vi "SMTP Email Command.vi"(4 "error in (no error)":errorcluster, 6 "command":string, 7 "smtp session":T1) -> (0 "error out":errorcluster, 1 "reply":string, 2 "reply code":i32, 3 "smtp session out":T1)   [LabVIEW 2011, in "NewNI_SMTPEmail.lvlib"]
doc: "General pupose VI that sends any kind of message (command) to the SMTP server using \"SMTP Session\", and recieves a string of reply (possibly multiline as specified in RFC821)."
uses:
  NewNI_SMTPEmail.lvlib
  SMTP Email Session.ctl
panel:
  in  "tcp connection":refnum<k5>
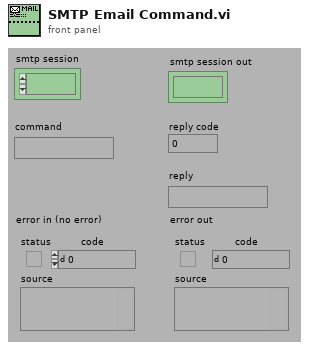
[diagram p1: front panel]
types:
  T1 = typedef "NewNI_SMTPEmail.lvlib/SMTP Email Session.ctl" = refnum<k1>
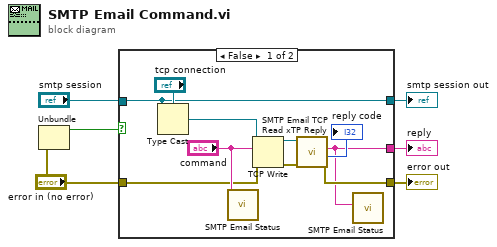
[diagram p0: block diagram]
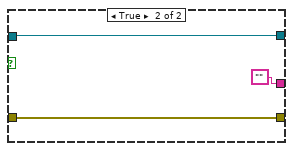
[diagram p2: hidden frame]
diagram:
  n1 = Unbundle("error in (no error)") -> ("status"=w2:bool)  [unwired: 2 out]
  n2 = case shown="False" w2 {
    tunnel: "smtp session" -> [w11 w19]
    tunnel: [w14 w17] -> w1
    tunnel: [w9 ""] -> w5
    tunnel: [w11 w19] -> w4
    tunnel: "error in (no error)" -> [w7 w17]
    frame False {
      n3 = Type Cast(type="tcp connection", x=w11) -> (*(type *) &x=w12:refnum<k5>)
      n4 = call "SMTP Email Status"("action string"="command") -> ()  [unwired: 2 in, 9 out]
      n5 = TCP Write(connection ID=w12, data in="command", error in (no error)=w7) -> (connection ID out=w15:refnum<k5>, error out=w16:errorcluster)  [unwired: 1 in, 1 out]
      n6 = call "SMTP Email TCP Read xTP Reply.vi"("error in (no error)"=w16, "buffered tcp connection"=w15) -> ("error out"=w14:errorcluster, "reply code"=→"reply code":i32, "reply string"=w9:string)  [unwired: 7 out]
      n7 = call "SMTP Email Status"("status string"=w9) -> ()  [unwired: 2 in, 9 out]
    }
    frame True {
    }
  }
  "error out" <- w1
  "reply" <- w5
  "smtp session out" <- w4
